vi "pulse Tx 16 spc.vi"(9 "enable line":bool=TRUE, 10 "take it!":bool, 11 "Cluster":T2={"PW"=0, "frequency shift"=0.0, "amp"=0.9999923706054688, "mode type"=enum."CW", "mode depth"=0, "mode filter"=0, "phase shift"=0.0, "pulse shape filter"=0}) -> (0 "output valid":bool, 1 "IQ out":T1[](array[typedef]), 2 "free dds":bool, 4 "frequncy":fxp<+/-,48,0>, 6 "phase":fxp<+/-,16,1>)   [LabVIEW 2021]
uses:
  Program Files/National Instruments/LabVIEW 2022/instr.lib/_niInstr/DSP/v1/Shared/Public/IQ Data.ctl
  Program Files/National Instruments/LabVIEW 2022/instr.lib/_niInstr/DSP/v1/Shared/niInstr DSP v1 Shared.lvlib
  Program Files/National Instruments/LabVIEW 2022/instr.lib/_niInstr/Basic Elements/v1/FPGA/niInstr Basic Elements v1 FPGA.lvlib
  <vilib>/rvi/FXPMathLib/FxpAdd/XNode/nifxpmath_Add.xnode
  <vilib>/rvi/FXPMathLib/sim/FxpSim.dll
  Program Files/National Instruments/LabVIEW 2022/instr.lib/_niInstr/Basic Elements/v1/FPGA/Private/Count Up U32.vi
  pulse_tx_vis/pdw.ctl
  pulse_tx_vis/mode_type.ctl
  Program Files/National Instruments/LabVIEW 2022/instr.lib/_niInstr/DSP/v1/FPGA/niInstr DSP v1 FPGA.lvlib
  <instrlib>/_niInstr/DSP/v1/FPGA/Public/Sub VIs/Frequency Shift/Frequency Shift - 16 spc.vi
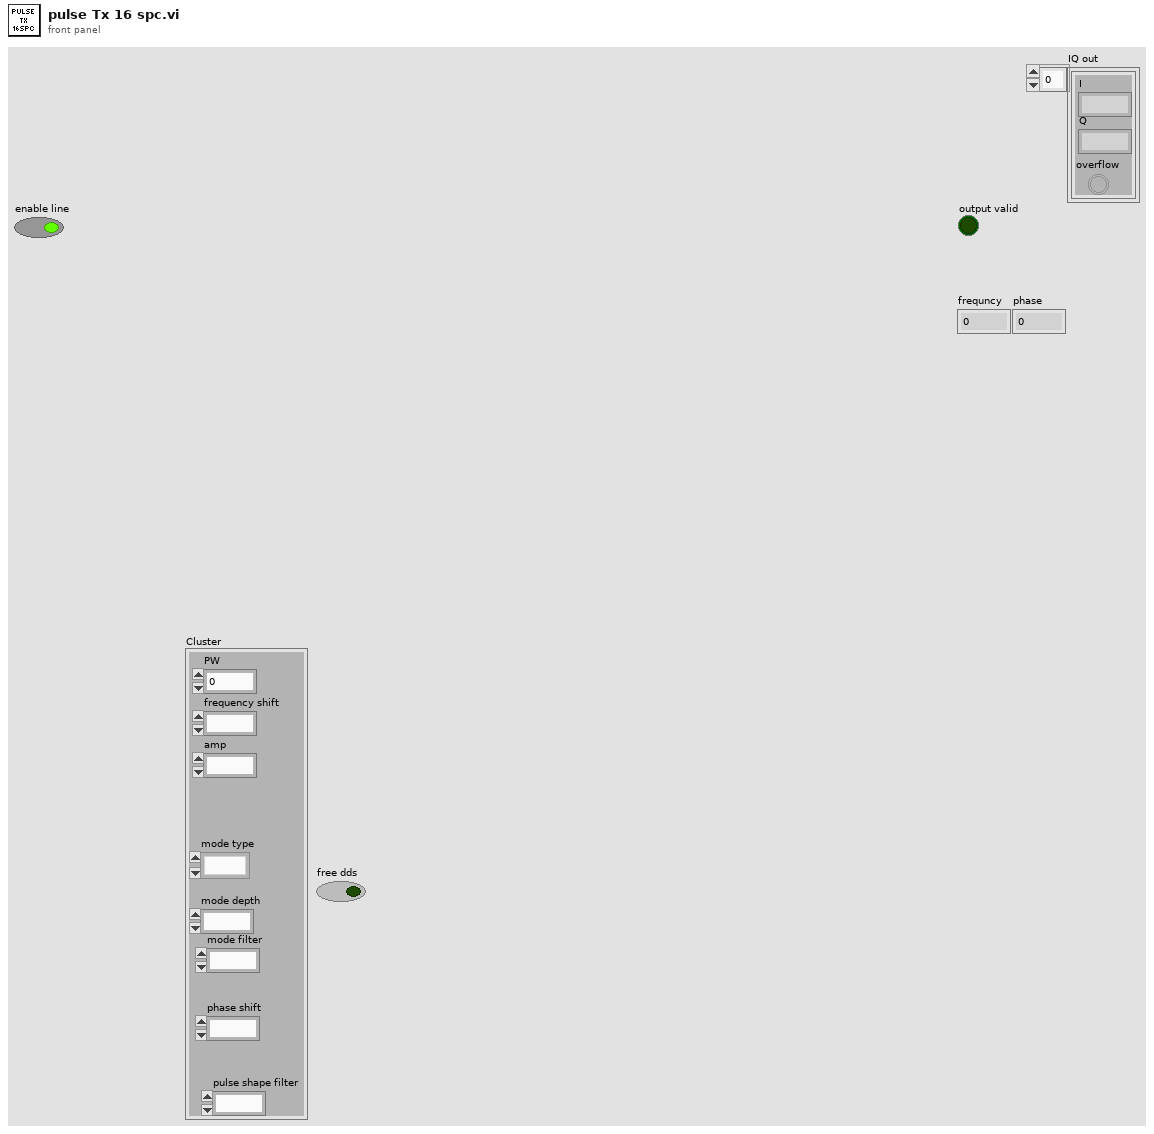
[diagram p1: front panel]
types:
  T1 = typedef "niInstr DSP v1 Shared.lvlib/IQ Data.ctl" = cluster{"I":fxp<+/-,18,1>, "Q":fxp<+/-,18,1>, "overflow":bool}
  T2 = typedef "pdw.ctl" = cluster{"PW":u32, "frequency shift":fxp<+/-,48,0>, "amp":fxp<+/-,18,1>, "mode type":T3, "mode depth":u32, "mode filter":u8, "phase shift":fxp<+/-,16,1>, "pulse shape filter":u8}
  T3 = typedef "mode_type.ctl" = enum8{"CW", "NC - CW", "NC - cw", "LFM", "BPSK", "QPSK"}
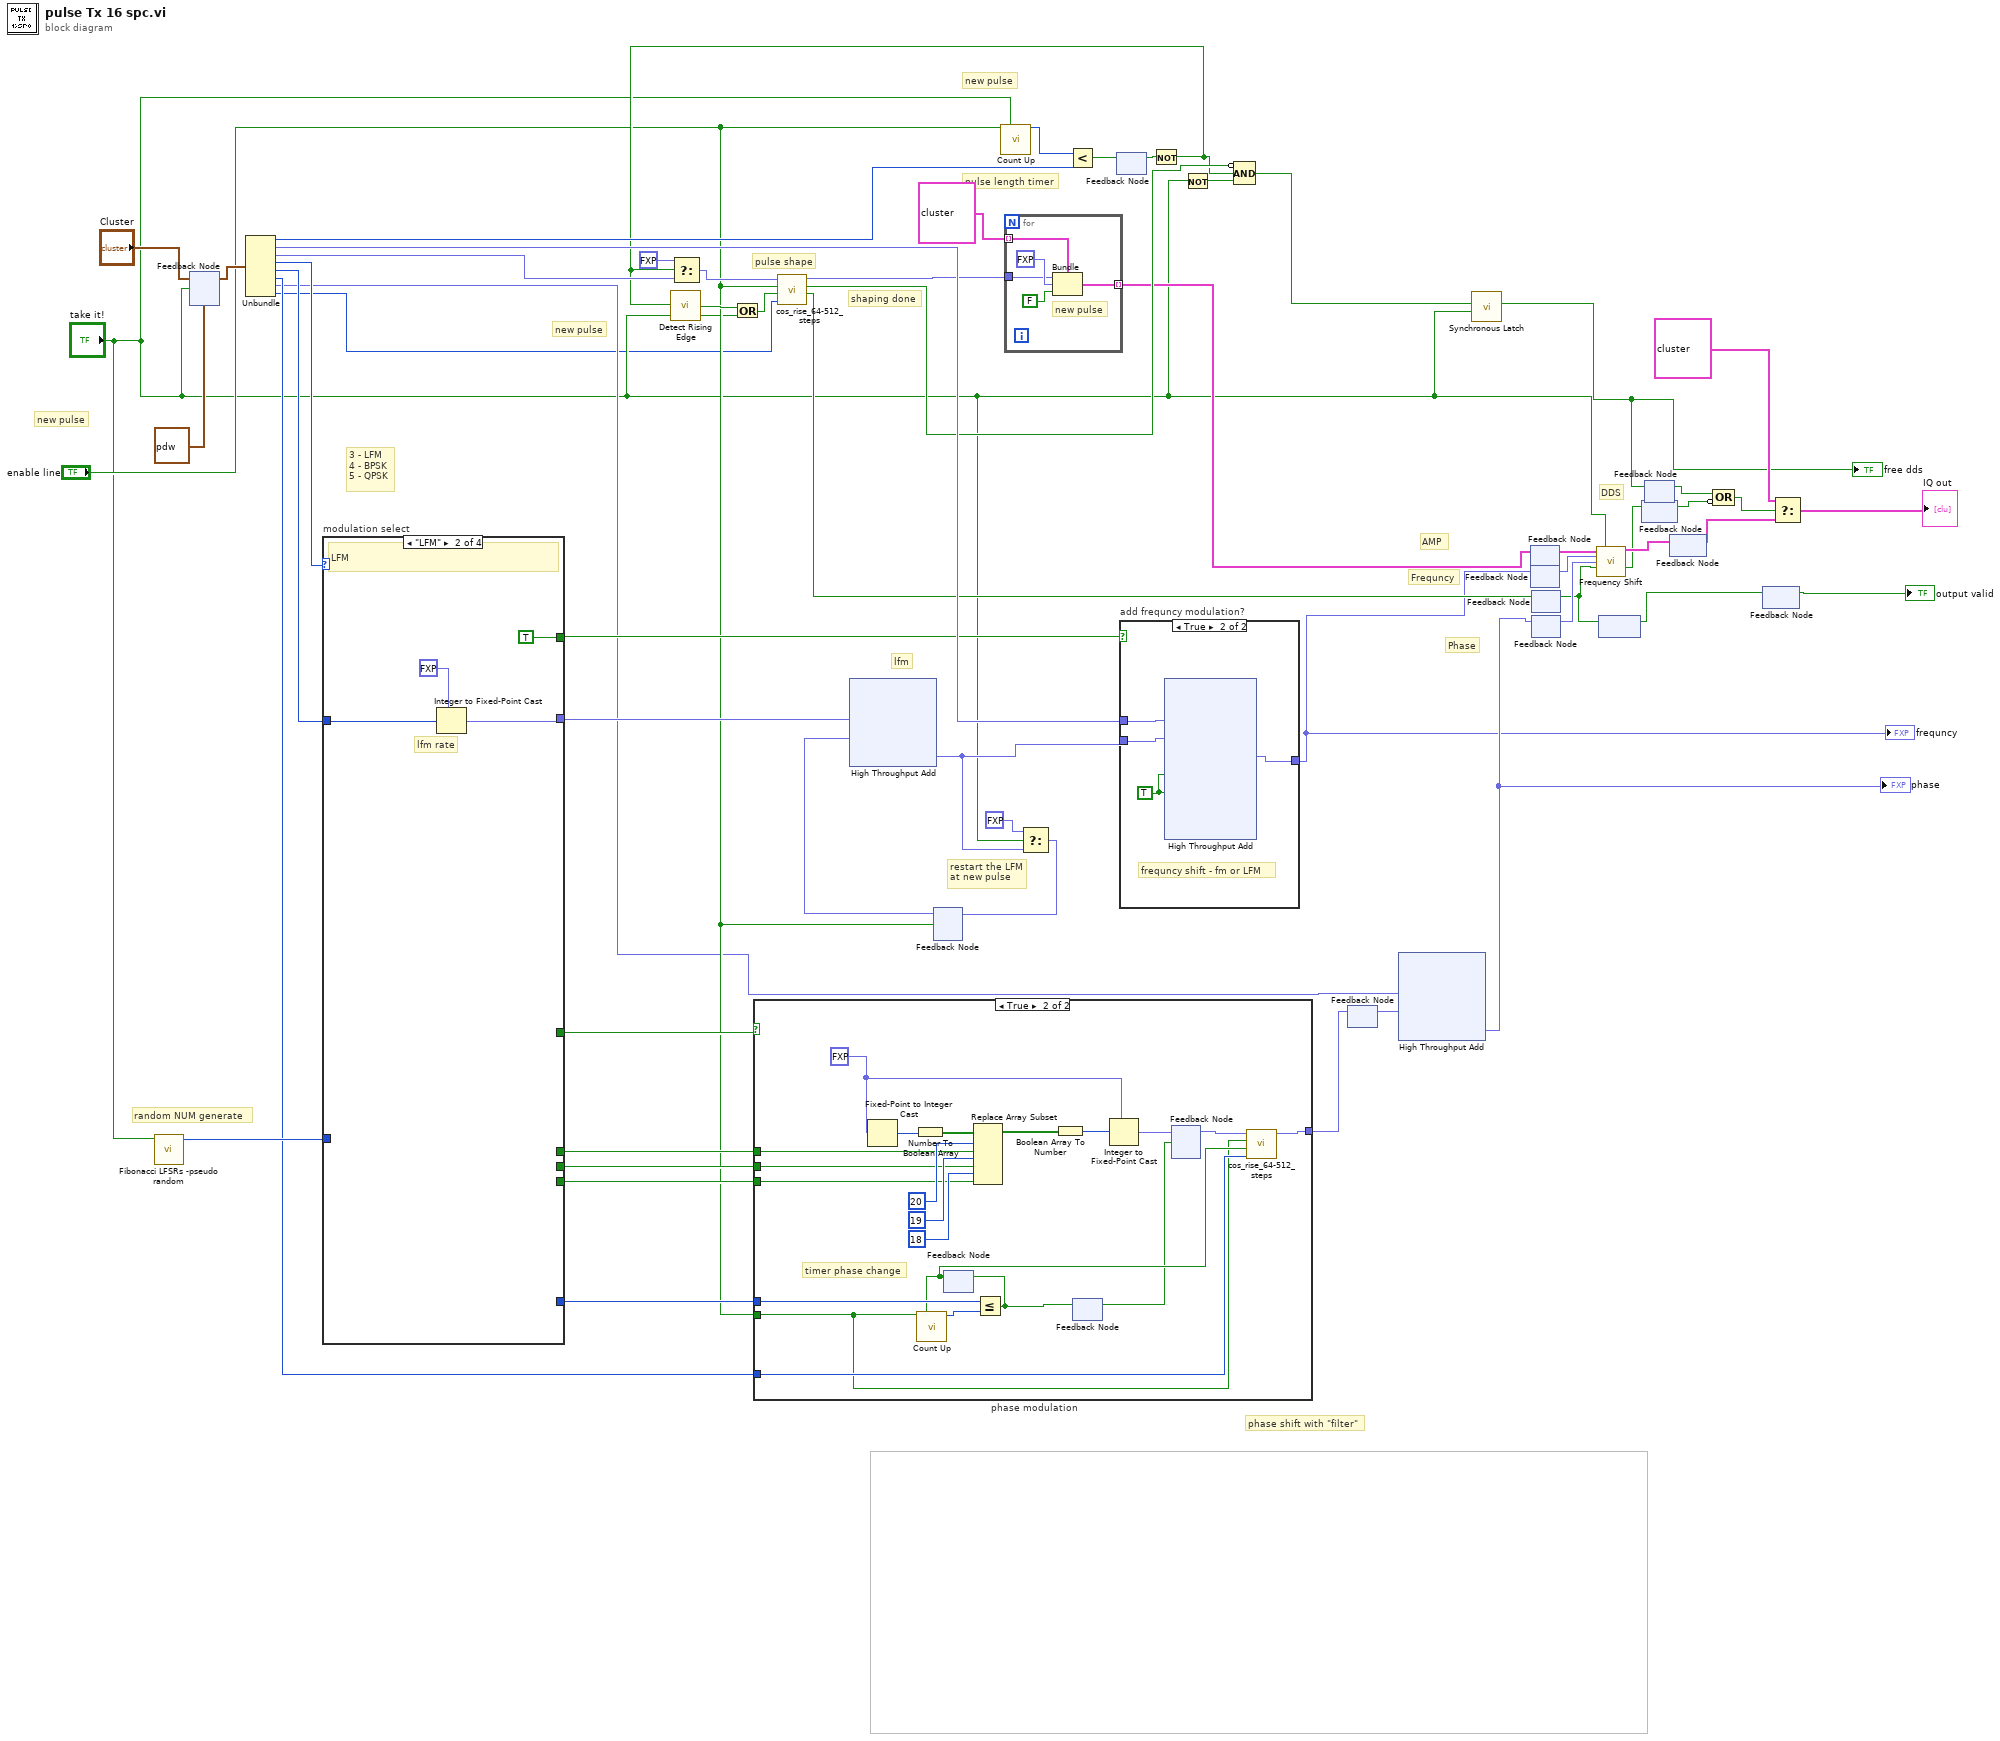
[diagram p0: block diagram]
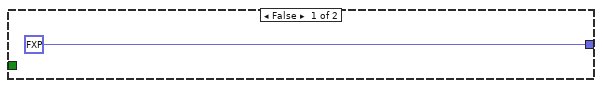
[diagram p2: hidden frame]
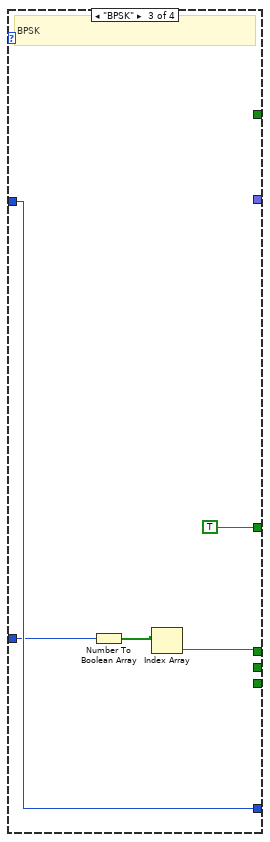
[diagram p5: hidden frame]
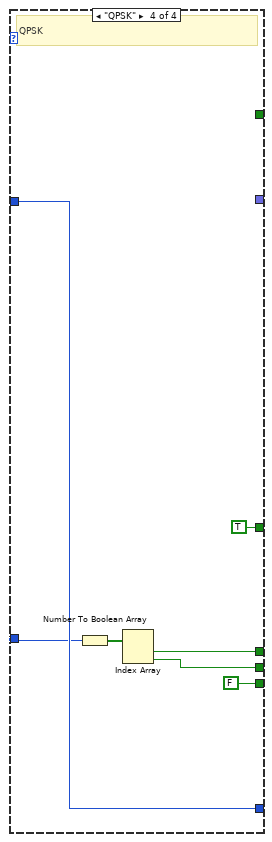
[diagram p6: hidden frame]
diagram:
  # "random NUM generate"
  # "phase shift with \"filter\""
  # "Phase"
  # "Frequncy"
  # "AMP"
  # "DDS"
  # "shaping done"
  # "3 - LFM\n4 - BPSK\n5 - QPSK"
  # "pulse length timer"
  # "restart the LFM\nat new pulse"
  # "lfm"
  # "pulse shape"
  # "new pulse"
  # "new pulse"
  # "new pulse"
  n1 = call "Fibonacci LFSRs -pseudo random.vi"("reset random"="take it!") -> ("rand number"=w33:u16)  [unwired: 10 in]
  n2 = feedback #1(T2 {"PW"=0, "frequency shift"=0.0, "amp"=0.9999923706054688, "mode type"=enum."CW", "mode depth"=0, "mode filter"=0, "phase shift"=0.0, "pulse shape filter"=0} ("Cluster")) -> (w57:T2)
  n3 = feedback-in #1("Cluster", "take it!") -> ()
  n4 = Unbundle(w57) -> ("PW"=w59:u32, "frequency shift"=w53:fxp<+/-,48,0>, "amp"=w36:fxp<+/-,18,1>, "mode type"=w54:T3, "mode depth"=w28:u32, "mode filter"=w27:u8, "phase shift"=w25:fxp<+/-,16,1>, "pulse shape filter"=w10:u8)
  n5 = case "modulation select" shown="\"LFM\"" w54 {
    tunnel: w28 -> [_ w62 w65 w70]
    tunnel: [_ w61 _ _] -> w50
    tunnel: [_ TRUE ("s") _ _] -> w47
    tunnel: [_ _ _ FALSE] -> w45
    tunnel: [_ _ _ w72] -> w44
    tunnel: [_ _ w67 w74] -> w43
    tunnel: [_ _ TRUE TRUE] -> w42
    tunnel: [_ _ w65 w70] -> w41
    tunnel: w33 -> [_ _ w64 w69]
    frame Default {
    }
    frame "LFM" {
      # "lfm rate"
      # "LFM"
      n6 = Integer to Fixed-Point Cast(fixed-point type=fxp<+,32,-16> 0.0, integer=w62) -> (fixed-point=w61:fxp<+,32,-16>)
    }
    frame "BPSK" {
      # "BPSK"
      n7 = Number To Boolean Array(number=w64) -> (Boolean array=w68:bool[])
      n8 = Index Array(array=w68) -> (element=w67:bool)  [unwired: 1 in]
    }
    frame "QPSK" {
      # "QPSK"
      n9 = Number To Boolean Array(number=w69) -> (Boolean array=w75:bool[])
      n10 = Index Array(array=w75) -> (element #1=w74:bool, element #2=w72:bool)  [unwired: 2 in]
    }
  }
  n11 = case "phase modulation" shown="True" w42 {
    tunnel: w45 -> [_ w89]
    tunnel: w44 -> [_ w88]
    tunnel: w43 -> [_ w87]
    tunnel: w41 -> [_ w85]
    tunnel: [fxp<+/-,16,1> 0.0 ("filter out") w82] -> w12
    tunnel: w27 -> [_ w80]
    tunnel: "enable line" -> [_ w79]
    frame False {
    }
    frame True {
      w91 = fxp<+/-,21,0> 0.0 ("phase")
      # "timer phase change"
      n12 = Fixed-Point to Integer Cast(1:w91) -> (0:w97:i32)
      n13 = Number To Boolean Array(number=w97) -> (Boolean array=w95:bool[])
      n14 = feedback #2() -> (w81:bool)  [unwired: 1 in]
      n15 = call-poly "Count Up.vi"("increment"=w79, "reset"=w81) -> ("count out"=w84:u32)  [unwired: 13 in]
      n16 = Replace Array Subset(array=w95, new element #1=w87, index #1=20 ("index"), new element #2=w88, index #2=19 ("index"), new element #3=w89, index #3=18 ("index")) -> (w90:bool[])
      n17 = Less Or Equal?(x=w85, y=w84) -> (x <= y?=w78:bool)
      n18 = feedback-in #2(w78) -> ()
      n19 = Boolean Array To Number(Boolean array=w90) -> (number=w96:u32)
      n20 = feedback-in #3(w78) -> ()
      n21 = feedback #3() -> (w77:bool)  [unwired: 1 in]
      n22 = Integer to Fixed-Point Cast(fixed-point type=w91, integer=w96) -> (fixed-point=w86:fxp<+/-,21,0>)
      n23 = feedback-in #4(w86, w77) -> ()
      n24 = feedback #4() -> (w83:fxp<+/-,21,0>)  [unwired: 1 in]
      n25 = call "cos_rise_64-512_steps.vi"("filter select"=w80, "new step"=w81, "run"=w79, "data in"=w83) -> ("data out"=w82:fxp<+/-,16,1>)  [unwired: 5 in, 2 out]
    }
  }
  n26 = feedback #5() -> (w49:fxp<+/-,48,0>)  [unwired: 1 in]
  n27 = xnode ("High Throughput Add")("x"=w50, "y"=w49) -> ("x+y"=w48:fxp<+/-,48,0>)
  n28 = call-poly "Count Up.vi"("increment"="enable line", "reset"="take it!") -> ("count out"=w40:u32)  [unwired: 13 in]
  n29 = Select(t=fxp<+/-,48,0> 0.0, s="take it!", f=w48) -> (s? t:f=w51:fxp<+/-,48,0>)
  n30 = feedback-in #5(w51, "enable line") -> ()
  n31 = Less?(x=w40, y=w59) -> (x < y?=w39:bool)
  n32 = feedback #6() -> (w38:bool)  [unwired: 1 in]
  n33 = feedback-in #6(w39) -> ()
  n34 = case "add frequncy modulation?" shown="True" w47 {
    tunnel: w53 -> [w98 w102]
    tunnel: w48 -> [_ w101]
    tunnel: [w98 w100] -> w22
    frame False {
    }
    frame True {
      w99 = TRUE ("input valid")
      # "frequncy shift - fm or LFM"
      n35 = xnode ("High Throughput Add")("x"=w102, "y"=w101, "input valid"=w99, "ready for output (T)"=w99) -> ("x+y"=w100:fxp<+/-,48,0>)  [unwired: 2 out]
    }
  }
  "frequncy" <- w22
  n36 = Not(x=w38) -> (.not. x?=w30:bool)
  n37 = call "Detect Rising Edge.vi"("signal"=w30) -> ("edge detected"=w29:bool)  [unwired: 14 in]
  n38 = Select(t=fxp<+/-,18,1> 0.0, s=w30, f=w36) -> (s? t:f=w35:fxp<+/-,18,1>)
  n39 = Or(x=w29, y="take it!") -> (x .or. y?=w31:bool)
  n40 = call "cos_rise_64-512_steps.vi"("filter select"=w10, "new step"=w31, "run"="enable line", "data in"=w35) -> ("output valid"=w23:bool, "steping"=w37:bool, "data out"=w32:fxp<+/-,16,1>)  [unwired: 5 in]
  n41 = for {
    tunnel: w32 -> [w105]
    tunnel: [w104] -> w21 mode=indexing
    tunnel: T1[] [{"I"=0.0, "Q"=0.0, "overflow"=FALSE}, {"I"=0.0, "Q"=0.0, "overflow"=FALSE}, {"I"=0.0, "Q"=0.0, "overflow"=FALSE}, {"I"=0.0, "Q"=0.0, "overflow"=FALSE}, {"I"=0.0, "Q"=0.0, "overflow"=FALSE}, {"I"=0.0, "Q"=0.0, "overflow"=FALSE}, {"I"=0.0, "Q"=0.0, "overflow"=FALSE}, {"I"=0.0, "Q"=0.0, "overflow"=FALSE}, {"I"=0.0, "Q"=0.0, "overflow"=FALSE}, {"I"=0.0, "Q"=0.0, "overflow"=FALSE}, {"I"=0.0, "Q"=0.0, "overflow"=FALSE}, {"I"=0.0, "Q"=0.0, "overflow"=FALSE}, {"I"=0.0, "Q"=0.0, "overflow"=FALSE}, {"I"=0.0, "Q"=0.0, "overflow"=FALSE}, {"I"=0.0, "Q"=0.0, "overflow"=FALSE}, {"I"=0.0, "Q"=0.0, "overflow"=FALSE}] ("t") -> [w103] mode=indexing
    # "new pulse"
    n42 = Bundle(cluster=w103, "I"=w105, "Q"=fxp<+/-,18,1> 0.0, "overflow"=FALSE ("input valid")) -> (w104:T1)
  }
  n43 = Not(x="take it!") -> (.not. x?=w56:bool)
  n44 = Compound Arithmetic op=AND(invert w37, w30, w56) -> (w55:bool)
  n45 = feedback-in #7(w12) -> ()
  n46 = feedback #7() -> (w11:fxp<+/-,16,1>)  [unwired: 1 in]
  n47 = xnode ("High Throughput Add")("x"=w25, "y"=w11) -> ("x+y"=w24:fxp<+/-,16,1>)
  "phase" <- w24
  n48 = call "Synchronous Latch.vi"("clear"="take it!", "set"=w55) -> ("out"=w2:bool)  [unwired: 9 in]
  "free dds" <- w2
  n49 = feedback #8() -> (w15:T1[])  [unwired: 1 in]
  n50 = feedback-in #8(w21) -> ()
  n51 = feedback #9() -> (w19:fxp<+/-,48,0>)  [unwired: 1 in]
  n52 = feedback-in #9(w22) -> ()
  n53 = feedback #10() -> (w7:bool)  [unwired: 1 in]
  n54 = feedback-in #10(w23) -> ()
  n55 = feedback-in #11(w24) -> ()
  n56 = feedback #11() -> (w18:fxp<+/-,16,1>)  [unwired: 1 in]
  n57 = call-poly <instrlib>:"Frequency Shift.vi"("data in"=w15, "reset"="take it!", "frequency shift"=w19, "phase"=w18, "input valid"=w7) -> ("data out"=w14:T1[], "output valid"=w4:bool)  [unwired: 7 in, 2 out]
  n58 = feedback #12() -> (w6:bool)  [unwired: 1 in]
  n59 = feedback-in #12(w7) -> ()
  n60 = feedback #13() -> (w3:bool)  [unwired: 1 in]
  n61 = feedback-in #13(w4) -> ()
  n62 = feedback #14() -> (w1:bool)  [unwired: 1 in]
  n63 = feedback-in #14(w2) -> ()
  n64 = feedback #15() -> (w13:T1[])  [unwired: 1 in]
  n65 = feedback-in #15(w14) -> ()
  n66 = Compound Arithmetic op=OR(w1, invert w3) -> (w9:bool)
  n67 = feedback #16() -> (→"output valid":bool)  [unwired: 1 in]
  n68 = feedback-in #16(w6) -> ()
  n69 = Select(t=T1[] [{"I"=0.0, "Q"=0.0, "overflow"=FALSE}, {"I"=0.0, "Q"=0.0, "overflow"=FALSE}, {"I"=0.0, "Q"=0.0, "overflow"=FALSE}, {"I"=0.0, "Q"=0.0, "overflow"=FALSE}, {"I"=0.0, "Q"=0.0, "overflow"=FALSE}, {"I"=0.0, "Q"=0.0, "overflow"=FALSE}, {"I"=0.0, "Q"=0.0, "overflow"=FALSE}, {"I"=0.0, "Q"=0.0, "overflow"=FALSE}, {"I"=0.0, "Q"=0.0, "overflow"=FALSE}, {"I"=0.0, "Q"=0.0, "overflow"=FALSE}, {"I"=0.0, "Q"=0.0, "overflow"=FALSE}, {"I"=0.0, "Q"=0.0, "overflow"=FALSE}, {"I"=0.0, "Q"=0.0, "overflow"=FALSE}, {"I"=0.0, "Q"=0.0, "overflow"=FALSE}, {"I"=0.0, "Q"=0.0, "overflow"=FALSE}, {"I"=0.0, "Q"=0.0, "overflow"=FALSE}], s=w9, f=w13) -> (s? t:f=→"IQ out":T1[])
